vi "Cycle.vi"(8 "error in (no error)":errorcluster, 11 "DotMappingExperiment In":refnum<class "DotMappingExperiment.lvclass">) -> (0 "error out":errorcluster, 3 "DotMappingExperiment Out":refnum<class "DotMappingExperiment.lvclass">)   [LabVIEW 2010]
uses:
  DotMappingExperiment.lvclass
panel:
  in  "Eye Params":dbl[](array[numeric])
  out "XY Graph":cluster{"horizontal":dbl[], "vertical":dbl[]}[](graph)
  out "ExperimentStats":T1
  in  "FixationRadius":dbl=50.0
  in  "RewardAmount":dbl=50.0
  in  "Timeouts":T2={"Intertrial"=1000.0, "AcquireFixation"=1000.0, "HoldFixation"=300.0, "DelayPeriod"=1000.0, "ResponsePeriod"=1000.0}
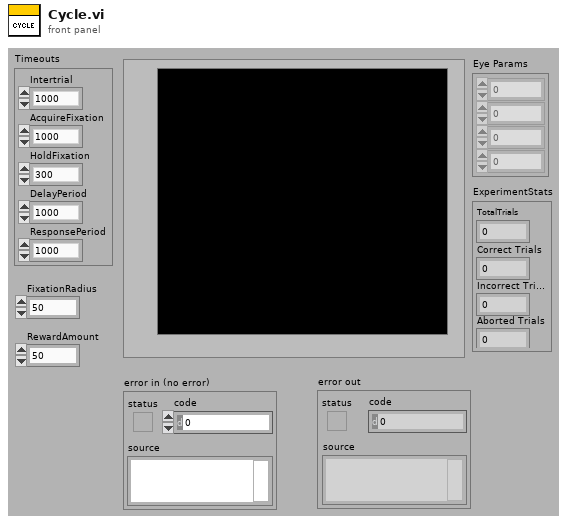
[diagram p1: front panel]
types:
  T1 = cluster{"TotalTrials":dbl, "Correct Trials":dbl, "Incorrect Trials":dbl, "Aborted Trials":dbl}
  T2 = cluster{"Intertrial":dbl, "AcquireFixation":dbl, "HoldFixation":dbl, "DelayPeriod":dbl, "ResponsePeriod":dbl}
  T3 = cluster{"TotalTrials":u32, "Correct Trials":u32, "Incorrect Trials":u32, "Aborted Trials":u32}
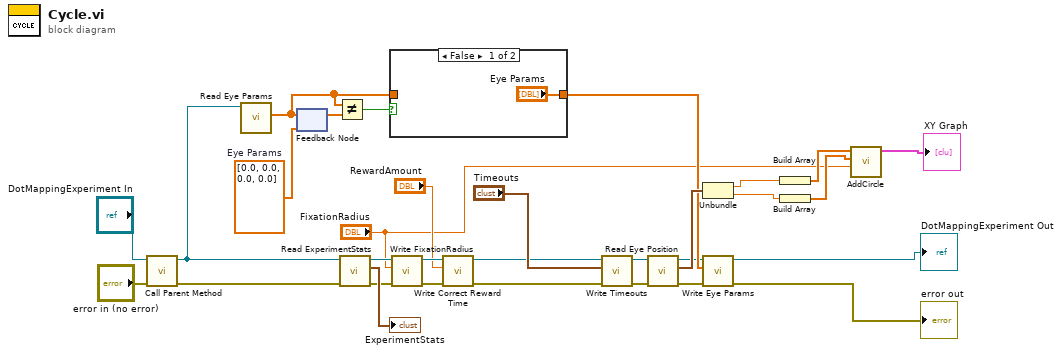
[diagram p0: block diagram]
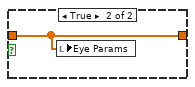
[diagram p2: hidden frame]
diagram:
  w23 = dbl[] [0.0, 0.0, 0.0, 0.0]  # Eye Params
  n1 = call-parent "Call Parent Method"("error in (no error)"="error in (no error)", "PassiveExperiment In"="DotMappingExperiment In") -> ("error out"=w9:errorcluster, "PassiveExperiment Out"=w3:refnum<class "DotMappingExperiment.lvclass">)  [unwired: 8 in]
  n2 = call-dynamic "Read Eye Params.vi"("TrialBasedExperiment in"=w3) -> ("Eye Params"=w24:dbl[])  [unwired: 8 in, 2 out]
  n3 = feedback #1(w23) -> (w21:dbl[])
  n4 = feedback-in #1(w24) -> ()
  n5 = Not Equal?(x=w24, y=w21) -> (x != y?=w22:bool)
  n6 = call-dynamic "Read ExperimentStats.vi"("error in (no error)"=w9, "TrialBasedExperiment in"=w3) -> ("error out"=w16:errorcluster, "ExperimentStats"=→"ExperimentStats":T3, "TrialBasedExperiment out"=w15:refnum<class "DotMappingExperiment.lvclass">)  [unwired: 7 in]
  n7 = case shown="False" w22 {
    tunnel: ["Eye Params" w33] -> w27
    tunnel: w24 -> [_ w33]
    frame False {
    }
    frame True {
      n8 = local write "Eye Params"(w33) -> ()
    }
  }
  n9 = call-dynamic "Write FixationRadius.vi"("error in (no error)"=w16, "FixationRadius"="FixationRadius", "MatlabExperiment in"=w15) -> ("error out"=w19:errorcluster, "MatlabExperiment out"=w18:refnum<class "DotMappingExperiment.lvclass">)  [unwired: 7 in]
  n10 = call-dynamic "Write Correct Reward Time.vi"("error in (no error)"=w19, "Correct Reward Time"="RewardAmount", "MatlabExperiment in"=w18) -> ("error out"=w4:errorcluster, "MatlabExperiment out"=w5:refnum<class "DotMappingExperiment.lvclass">)  [unwired: 7 in]
  n11 = call-dynamic "Write Timeouts.vi"("error in (no error)"=w4, "Timeouts"="Timeouts", "TrialBasedExperiment in"=w5) -> ("error out"=w2:errorcluster, "TrialBasedExperiment out"=w29:refnum<class "DotMappingExperiment.lvclass">)  [unwired: 7 in]
  n12 = call-dynamic "Read Eye Position.vi"("error in (no error)"=w2, "TrialBasedExperiment in"=w29) -> ("error out"=w26:errorcluster, "Eye Position"=w28:cluster{"Horizontal":dbl, "Vertical":dbl}, "TrialBasedExperiment out"=w25:refnum<class "DotMappingExperiment.lvclass">)  [unwired: 7 in]
  n13 = Unbundle(w28) -> ("Horizontal"=w14:dbl, "Vertical"=w13:dbl)
  n14 = call-dynamic "Write Eye Params.vi"("error in (no error)"=w26, "Eye Params"=w27, "TrialBasedExperiment in"=w25) -> ("error out"=→"error out":errorcluster, "TrialBasedExperiment out"=→"DotMappingExperiment Out":refnum<class "DotMappingExperiment.lvclass">)  [unwired: 7 in]
  n15 = Build Array(w14) -> (w12:dbl[])
  n16 = Build Array(w13) -> (w11:dbl[])
  n17 = call "AddCircle.vi"("radius"="FixationRadius", "vertical"=w11, "horizontal"=w12) -> ("output"=→"XY Graph":cluster{"horizontal":dbl[], "vertical":dbl[]}[])  [unwired: 8 in]
